vi "Generate-c.vi"(0 "Stop":bool) -> ()   [LabVIEW 2020]
uses:
  Typedefs/Stop cases.ctl
  Queue/Typedefs/Operations.ctl
panel:
  out "Error out":errorcluster
  in  "Error in":errorcluster
  # "GENERATE"
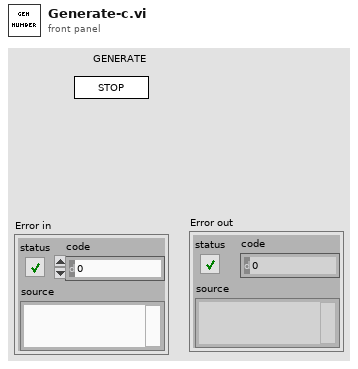
[diagram p1: front panel]
types:
  T1 = typedef "Operations.ctl" = enum16{"Initialize", "Enqueue", "Dequeue", "Sum"}
  T2 = typedef "Stop cases.ctl" = enum16{"Initialize", "Write", "Stop"}
  T3 = enum32{"Bad", "Idle", "Run top level", "Running"}
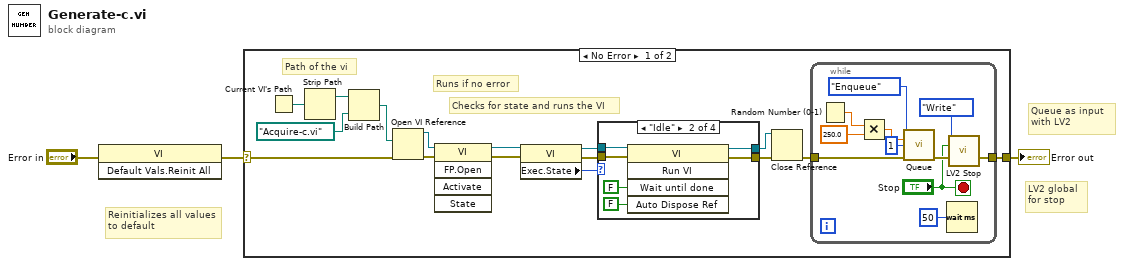
[diagram p0: block diagram]
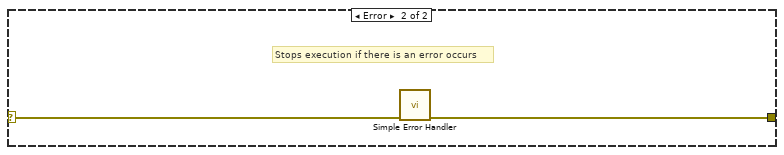
[diagram p5: hidden frame]
diagram:
  # "LV2 global \nfor stop"
  # "Queue as input \nwith LV2"
  # "Reinitializes all values\nto default"
  n1 = invoke class="VI" method="Default Vals.Reinit All"(error in="Error in") -> (error out=w2:errorcluster)  [unwired: 2 in, 2 out]
  n2 = case shown="No Error" w2 {
    selector: w2 -> [w13 w44]
    tunnel: [w4 w43] -> w3
    frame No Error {
      # "Checks for state and runs the VI"
      # "Runs if no error"
      # "Path of the vi"
      n3 = Current VI's Path() -> (path=w19:path)
      n4 = Strip Path(path=w19) -> (stripped path=w18:path)  [unwired: 1 out]
      n5 = Build Path(base path=w18, name or relative path=path "Acquire-c.vi") -> (appended path=w16:path)
      n6 = Open VI Reference(vi path=w16, error in (no error)=w13) -> (vi reference=w14:refnum<vi>, error out=w15:errorcluster)  [unwired: 4 in]
      n7 = invoke class="VI" method="FP.Open"(reference=w14, error in=w15) -> (reference out=w12:refnum<vi>, error out=w10:errorcluster)  [unwired: 3 in, 3 out]
      n8 = property class="VI"(reference=w12, error in=w10) -> (reference out=w11:refnum<vi>, error out=w9:errorcluster, "Exec.State"=w8:T3)
      n9 = case shown="\"Idle\"" w8 {
        tunnel: w11 -> [w20 w27 w29 w31]
        tunnel: w9 -> [w21 w26 w28 w30]
        tunnel: [w21 w23 w28 w30] -> w7
        tunnel: [w20 w22 w29 w31] -> w6
        frame "Bad" {
        }
        frame "Idle" {
          n10 = invoke class="VI" method="Run VI"(reference=w27, error in=w26, "Wait until done"=FALSE ("Wait Until Done"), "Auto Dispose Ref"=FALSE ("Auto Dispose Reference")) -> (reference out=w22:refnum<vi>, error out=w23:errorcluster)  [unwired: 1 in, 3 out]
        }
        frame "Run top level" {
        }
        frame "Running" {
        }
      }
      n11 = Close Reference(reference=w6, error in (no error)=w7) -> (error out=w5:errorcluster)
      n12 = while {
        tunnel: w5 -> [w39]
        tunnel: [w37] -> w4
        stop <- "Stop" stop-if-true
        n13 = Random Number (0-1)() -> (number: 0 to 1=w42:dbl)
        n14 = Multiply(x=w42, y=250.0) -> (x*y=w40:dbl)
        n15 = call "Queue.vi"("Operation"=Operations."Enqueue", "Enqueue"=w40, "Size"=1, "Error in"=w39) -> ("Error out"=w38:errorcluster)  [unwired: 6 in, 5 out]
        n16 = Wait (ms)(milliseconds to wait=u32 50) -> ()  [unwired: 1 out]
        n17 = call "LV2 Stop.vi"("Operation"=Stop_cases."Write", "Stop"="Stop", "Error in"=w38) -> ("Error out"=w37:errorcluster)  [unwired: 11 in, 1 out]
      }
    }
    frame Error {
      # "Stops execution if there is an error occurs"
      n18 = call <vilib>:"Simple Error Handler.vi"("error in (no error)"=w44) -> ("error out"=w43:errorcluster)  [unwired: 4 in, 4 out]
    }
  }
  "Error out" <- w3
